vi "Read Unit Config File.vi"(1 "Unit Config File Path":path) -> (0 "Unit Config File":T1 {"Section"."Conversion Table"."Zero" format="%.2f"; "Section"."Conversion Table"."Span" format="%.2f"})   [LabVIEW 2023]
uses:
  <vilib>/Utility/config.llb/Read Key (String).vi
  <vilib>/Utility/config.llb/NI_LVConfig.lvlib
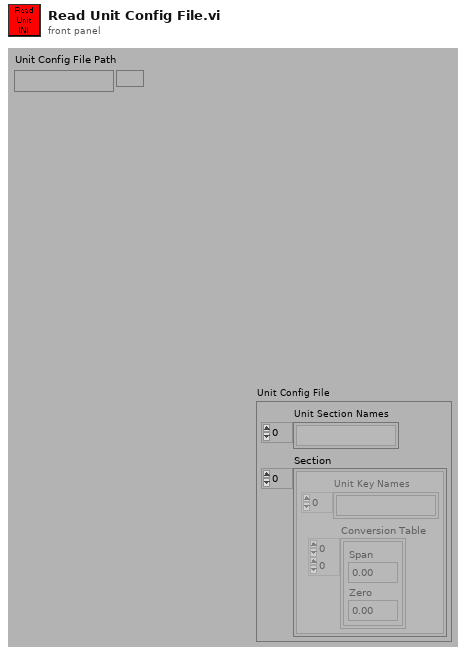
[diagram p1: front panel]
types:
  T1 = cluster{"Unit Section Names":string[], "Section":cluster{"Unit Key Names":string[], "Conversion Table":cluster{"Span":dbl, "Zero":dbl}[][]}[]}
  T2 = typedef "NI_LVConfig.lvlib/Config Data RefNum.ctl" = refnum<k1>
  T3 = cluster{"key names":string[], "Conversion Factors":cluster{"Span":dbl, "Zero":dbl}[][]}
  T4 = cluster{"section names":string[], cluster{"key names":string[], "Conversion Factors":cluster{"Span":dbl, "Zero":dbl}[][]}[]}
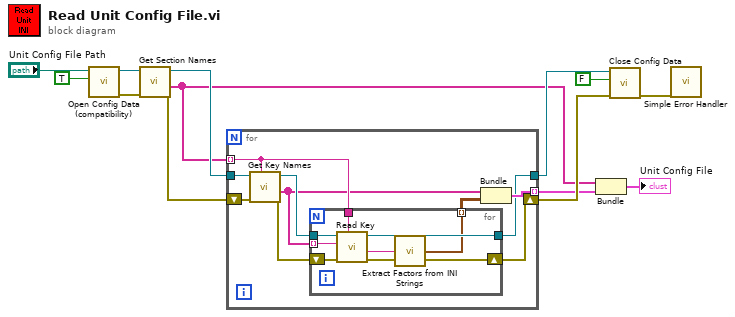
[diagram p0: block diagram]
diagram:
  n1 = call <vilib>:"Open Config Data (compatibility).vi"("create file if necessary (T)"=TRUE ("create file if necessary? (T)"), "configuration file path"="Unit Config File Path") -> ("error out"=w10:errorcluster, "refnum"=w11:T2)  [unwired: 7 in, 1 out]
  n2 = call <vilib>:"Get Section Names.vi"("error in (no error)"=w10, "refnum"=w11) -> ("error out"=w6:errorcluster, "section names"=w3:string[], "refnum out"=w8:T2)  [unwired: 7 in]
  n3 = for {
    tunnel: w3 -> [w18] mode=indexing
    tunnel: w8 -> [w23]
    tunnel: [w16] -> w7
    tunnel: [w22] -> w4 mode=indexing
    shift-right: [w15] -> w5
    shift-left: w6 -> [w21]
    n4 = call <vilib>:"Get Key Names.vi"("section"=w18, "error in (no error)"=w21, "refnum"=w23) -> ("error out"=w20:errorcluster, "key names"=w17:string[], "refnum out"=w19:T2)  [unwired: 5 in, 1 out]
    n5 = for {
      shift-right: [w30] -> w15
      shift-left: w20 -> [w31]
      tunnel: w19 -> [w29]
      tunnel: w18 -> [w28]
      tunnel: w17 -> [w27] mode=indexing
      tunnel: [w26] -> w16
      tunnel: [w24] -> w14 mode=indexing
      n6 = call-poly <vilib>:"Read Key.vi"("section"=w28, "error in (no error)"=w31, "key"=w27, "refnum"=w29) -> ("error out"=w30:errorcluster, "value"=w25:string, "refnum out"=w26:T2)  [unwired: 4 in, 1 out]
      n7 = call "Extract Factors from INI Strings.vi"("String"=w25) -> ("Conversion Factors"=w24:cluster{"Span":dbl, "Zero":dbl}[])
    }
    n8 = Bundle("key names"=w17, "Conversion Factors"=w14) -> (w22:T3)  [unwired: 1 in]
  }
  n9 = Bundle("section names"=w3, w4) -> (→"Unit Config File":T4)  [unwired: 1 in]
  n10 = call <vilib>:"Close Config Data.vi"("error in (no error)"=w5, "write file if changed (T)"=FALSE ("write configuration file? (T)"), "refnum"=w7) -> ("error out"=w9:errorcluster)  [unwired: 7 in, 1 out]
  n11 = call <vilib>:"Simple Error Handler.vi"("error in (no error)"=w9) -> ()  [unwired: 4 in, 5 out]
